vi "CreateProtectedEvents.vi"(8 "error in (no error)":errorcluster, 11 "0MQ_Server":refnum<class "0MQ_Server.lvclass">) -> (0 "error out":errorcluster, 3 "0MQ_Server out":refnum<class "0MQ_Server.lvclass">)   [LabVIEW 2016, in "0MQ_Server.lvclass"]
doc: "JKI State Machine Objects (SMO) 1.0.0.7\nJKI - JKI\nCopyright (c) 2016, JKI"
uses:
  0MQ_Server.lvclass
  0MQ_Server.lvclass/0MQ_Server.ctl
  <vilib>/JKI/JKI SMO/SMO/SMO.lvclass
panel:
  # "For instructions on how to use the JKI State Machine Objects, examples and video tutorials, visit:\nhttp://jki.net/state-machine-objects/\n\nJKI State Machine Objects™\nhttp://jki.net/state-machine-objects/\nCopyright (C) 2005-2015, JKI <info@jki.net>\nALL RIGHTS RESERVED"
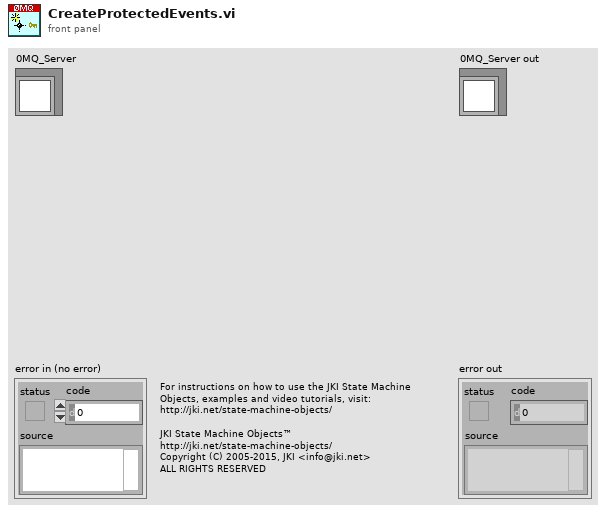
[diagram p1: front panel]
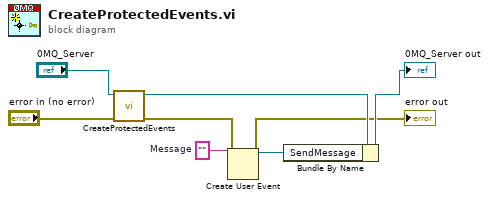
[diagram p0: block diagram]
diagram:
  w4 = ""  # Message
  n1 = call-parent "CreateProtectedEvents.vi"("error in (no error)"="error in (no error)", "SMO"="0MQ_Server") -> ("error out"=w2:errorcluster, "SMO out"=w6:refnum<class "0MQ_Server.lvclass">)  [unwired: 8 in]
  n2 = Create User Event(user event datatype=w4, error in=w2) -> (user event=w3:refnum<user-event>, error out=→"error out":errorcluster)
  n3 = Bundle By Name(cluster=w6, "SendMessage"=w3) -> (→"0MQ_Server out":refnum<class "0MQ_Server.lvclass">)
